vi "Gearbox set.vi"(8 "error in":errorcluster, 10 "Gearbox Speed":dbl, 11 "Gearbox Motors":T1) -> (0 "error out":errorcluster, 3 "Gearbox Motors dev rev":T1)   [LabVIEW 2013]
uses:
  GearBox Typedef.ctl
  <vilib>/Rock Robotics/WPI/MotorControl/WPI_MotorControlDeviceRef.ctl
  <vilib>/Rock Robotics/SystemInterfaces/Typedef/FPGA_TypedefDigitalModule.ctl
  <vilib>/Rock Robotics/SystemInterfaces/DIO/FPGA_DIOPWMChannel.ctl
  <vilib>/Rock Robotics/WPI/PWM/WPI_PWMDeadband.ctl
  <vilib>/Rock Robotics/WPI/CAN/Jaguar/SubVIs/WPI_CANJaguar_ControlMode.ctl
  <vilib>/Rock Robotics/WPI/PWM/WPI_PWMTransform_ConPane.ctl
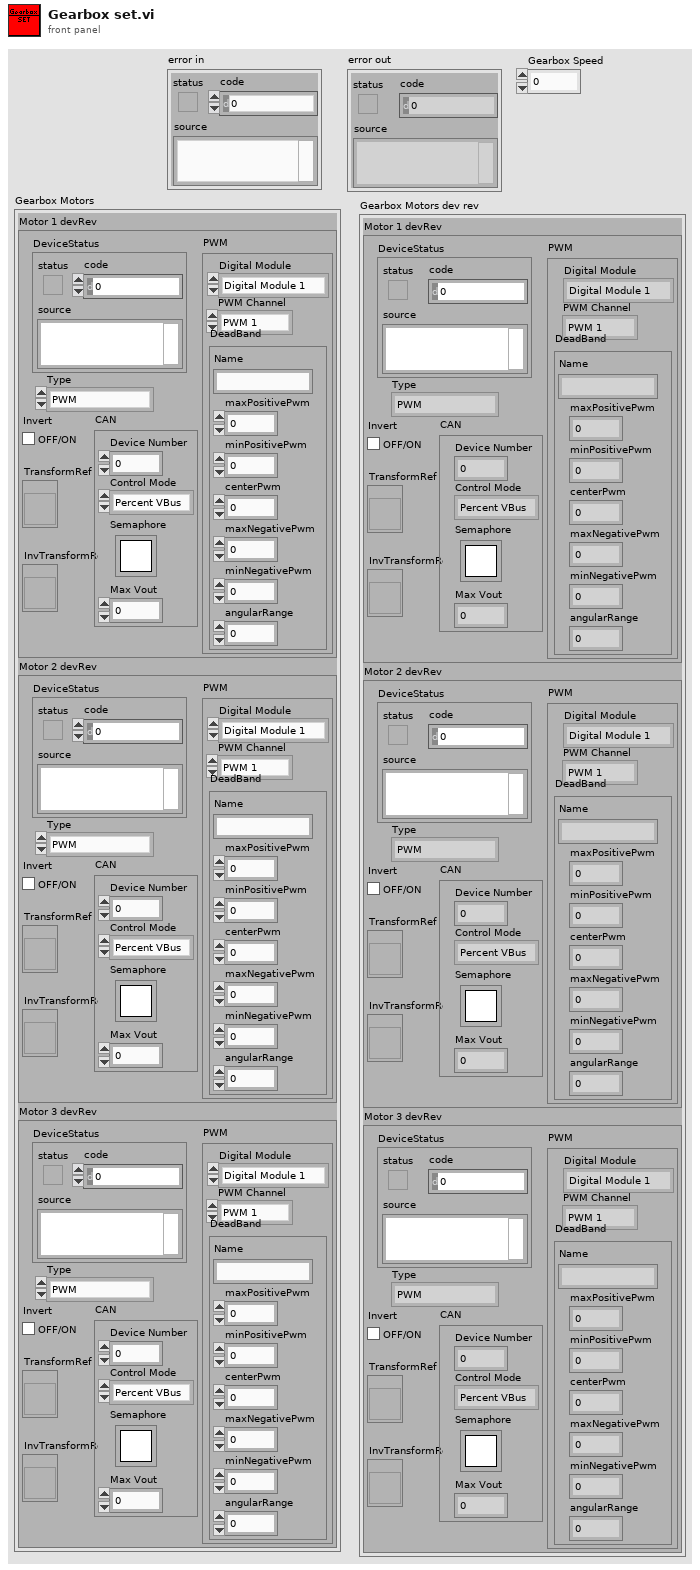
[diagram p1: front panel]
types:
  T1 = typedef "GearBox Typedef.ctl" = cluster{"Motor 1 devRev":T2, "Motor 2 devRev":T2, "Motor 3 devRev":T2}
  T2 = typedef "WPI_MotorControlDeviceRef.ctl" = cluster{"DeviceStatus":errorcluster, "Type":enum16{"PWM", "CAN"}, "PWM":cluster{"Digital Module":T3, "PWM Channel":T4, "DeadBand":T5}, "CAN":cluster{"Device Number":u8, "Control Mode":T6, "Semaphore":T7, "Max Vout":dbl}, "Invert":bool, "TransformRef":T8, "InvTransformRef":T8}
  T3 = typedef "FPGA_TypedefDigitalModule.ctl" = enum16{"Digital Module 1", "Digital Module 2"}
  T4 = typedef "FPGA_DIOPWMChannel.ctl" = enum8{"PWM 1", "PWM 2", "PWM 3", "PWM 4", "PWM 5", "PWM 6", "PWM 7", "PWM 8", "PWM 9", "PWM 10", "Invalid"}
  T5 = typedef "WPI_PWMDeadband.ctl" = cluster{"Name":string, "maxPositivePwm":i32, "minPositivePwm":i32, "centerPwm":i32, "maxNegativePwm":i32, "minNegativePwm":i32, "angularRange":u16}
  T6 = typedef "WPI_CANJaguar_ControlMode.ctl" = enum8{"Percent VBus", "Current", "Speed", "Position", "Voltage"}
  T7 = typedef "Semaphore RefNum" = refnum<k1>
  T8 = typedef "WPI_PWMTransform_ConPane.ctl" = refnum<vi>
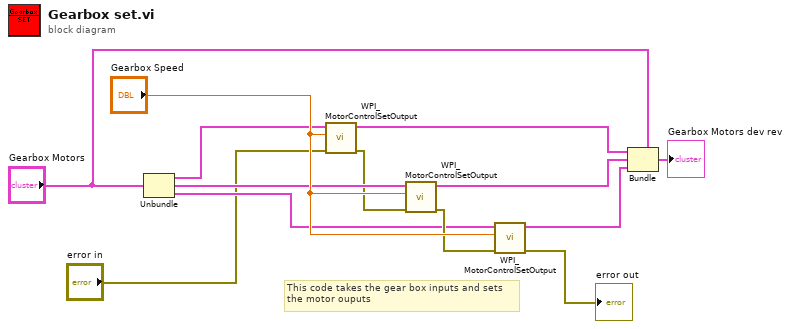
[diagram p0: block diagram]
diagram:
  # "This code takes the gear box inputs and sets\nthe motor ouputs"
  n1 = Unbundle("Gearbox Motors") -> ("Motor 1 devRev"=w8:T2, "Motor 2 devRev"=w10:T2, "Motor 3 devRev"=w11:T2)
  n2 = call <vilib>:"WPI_MotorControlSetOutput.vi"("error in (no error)"="error in", "Output"="Gearbox Speed", "MotorControlDevRef"=w8) -> ("error out"=w9:errorcluster, "MotorControlDevRef"=w5:T2)  [unwired: 6 in, 1 out]
  n3 = call <vilib>:"WPI_MotorControlSetOutput.vi"("error in (no error)"=w9, "Output"="Gearbox Speed", "MotorControlDevRef"=w10) -> ("error out"=w12:errorcluster, "MotorControlDevRef"=w4:T2)  [unwired: 6 in, 1 out]
  n4 = call <vilib>:"WPI_MotorControlSetOutput.vi"("error in (no error)"=w12, "Output"="Gearbox Speed", "MotorControlDevRef"=w11) -> ("error out"=→"error out":errorcluster, "MotorControlDevRef"=w3:T2)  [unwired: 6 in, 1 out]
  n5 = Bundle(cluster="Gearbox Motors", "Motor 1 devRev"=w5, "Motor 2 devRev"=w4, "Motor 3 devRev"=w3) -> (→"Gearbox Motors dev rev":T1)
